vi "ReadData.vi"(8 "Error In":errorcluster, 11 "reference in":refnum<class "EncryptedFileDataSource.lvclass">) -> (0 "Error Out":errorcluster, 2 "Return(STRING)":string, 3 "reference in":refnum<class "EncryptedFileDataSource.lvclass">)   [LabVIEW 2020, in "EncryptedFileDataSource.lvclass"]
uses:
  EncryptedFileDataSource.lvclass
  FileDataSource_class/FileDataSource.lvclass
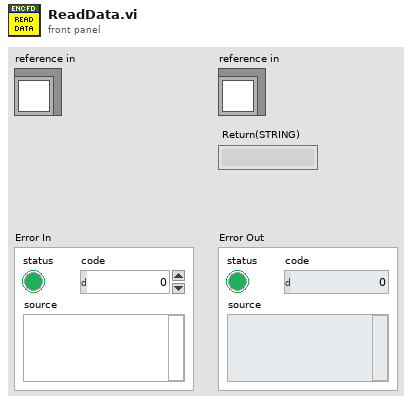
[diagram p1: front panel]
types:
  T1 = typedef "EncryptedFileDataSource.lvclass/ObjectAttributes.ctl" = cluster{"EncryptionType":T2}
  T2 = typedef "EncryptedFileDataSource.lvclass/EncryptionType.ctl" = enum16{"Type 1", "Type 2"}
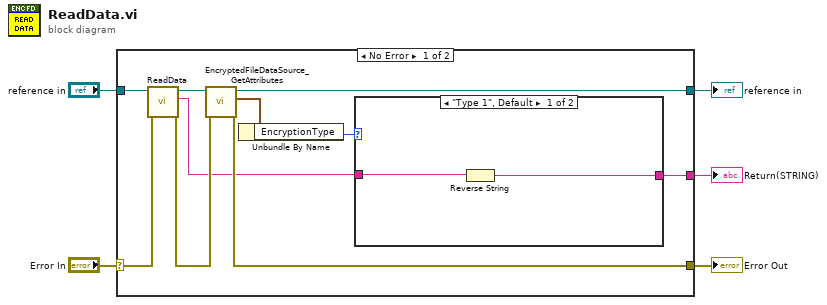
[diagram p0: block diagram]
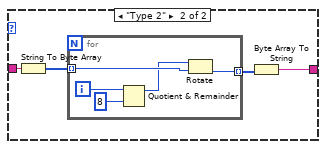
[diagram p2: hidden frame]
diagram:
  n1 = case shown="No Error" "Error In" {
    selector: "Error In" -> [w10 w28]
    tunnel: [w14 w28] -> w4
    tunnel: [w13 w27] -> w2
    tunnel: "reference in" -> [w12 w27]
    tunnel: [w6 _] -> w1
    frame No Error {
      n2 = call-parent "ReadData.vi"("Error In"=w10, "reference in"=w12) -> ("Error Out"=w9:errorcluster, "Return(STRING)"=w7:string, "reference out"=w11:refnum<class "EncryptedFileDataSource.lvclass">)  [unwired: 7 in]
      n3 = call "EncryptedFileDataSource_GetAttributes.vi"("error in (no error)"=w9, "reference in"=w11) -> ("error out"=w14:errorcluster, "Data"=w15:T1, "reference out"=w13:refnum<class "EncryptedFileDataSource.lvclass">)  [unwired: 6 in, 1 out]
      n4 = Unbundle By Name(w15) -> ("EncryptionType"=w8:T2)
      n5 = case shown="\"Type 1\", Default" w8 {
        tunnel: w7 -> [w17 w19]
        tunnel: [w16 w18] -> w6
        frame "Type 1", Default {
          n6 = Reverse String(1:w17) -> (0:w16:string)
        }
        frame "Type 2" {
          n7 = String To Byte Array(string=w19) -> (unsigned byte array=w20:u8[])
          n8 = for {
            tunnel: w20 -> [w24] mode=indexing
            tunnel: [w23] -> w21 mode=indexing
            i -> [w26]
            n9 = Quotient & Remainder(x=w26, y=8) -> (x-y*floor(x/y)=w22:i32)  [unwired: 1 out]
            n10 = Rotate(1:w24, 2:w22) -> (0:w23:u8)
          }
          n11 = Byte Array To String(unsigned byte array=w21) -> (string=w18:string)
        }
      }
    }
    frame Error {
    }
  }
  "Error Out" <- w4
  "reference in" <- w2
  "Return(STRING)" <- w1
